vi "Init.vi"(8 "error in (no error)":errorcluster, 11 "bt_System in":refnum<class "bt_System.lvclass">) -> (0 "error out":errorcluster, 3 "bt_System out":refnum<class "bt_System.lvclass">)   [LabVIEW 2021, in "BT.lvlib" / "bt_System.lvclass"]
uses:
  bt_System.lvclass
  bt_System.lvclass/bt_System.ctl
  Support/Execution Engine.vi
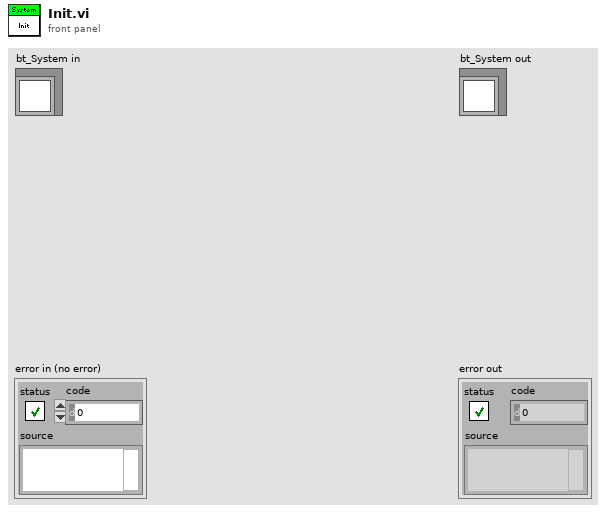
[diagram p1: front panel]
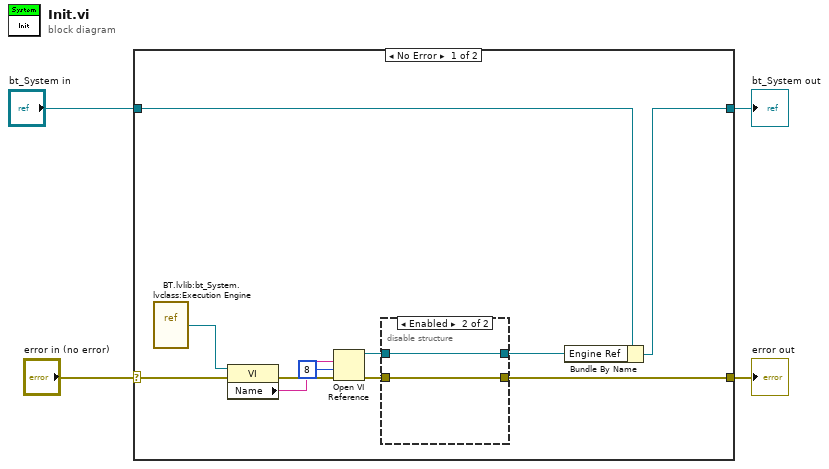
[diagram p0: block diagram]
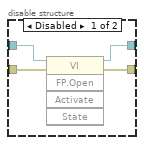
[diagram p2: hidden frame]
diagram:
  n1 = case shown="No Error" "error in (no error)" {
    selector: "error in (no error)" -> [w14 w23]
    tunnel: [w5 w23] -> w3
    tunnel: [w10 w22] -> w1
    tunnel: "bt_System in" -> [w11 w22]
    frame No Error {
      n2 = vi-ref "BT.lvlib:bt_System.lvclass:Execution Engine.vi"() -> (w13:refnum<vi>)
      n3 = property class="VI"(reference=w13, error in=w14) -> (error out=w15:errorcluster, "Name"=w12:string)  [unwired: 1 out]
      n4 = Open VI Reference(vi path=w12, options=8, error in (no error)=w15) -> (vi reference=w8:refnum<vi>, error out=w7:errorcluster)  [unwired: 3 in]
      n5 = disable-structure shown="Enabled" {
        disable-tunnel: w8 -> [w19 w21]
        disable-tunnel: w7 -> [w18 w20]
        disable-tunnel: [w17 w21] -> w6
        disable-tunnel: [w16 w20] -> w5
        frame Disabled {
          n6 = invoke class="VI" method="FP.Open"(reference=w19, error in=w18) -> (reference out=w17:refnum<vi>, error out=w16:errorcluster)  [unwired: 3 in, 3 out]
        }
        frame Enabled {
        }
      }
      n7 = Bundle By Name(cluster=w11, "Engine Ref"=w6) -> (w10:refnum<class "bt_System.lvclass">)
    }
    frame Error {
    }
  }
  "error out" <- w3
  "bt_System out" <- w1
